vi "CU_RatingVoting.vi"(8 "Classification Distribution":i32[][][](array[numeric]), 11 "IndicatorMatrix":dbl[][](array[numeric])) -> (3 "Class Index":i32)   [LabVIEW 2016, in "Classifier.lvlib"]
uses:
  <vilib>/Analysis/baseanly.llb/A x Vector.vi
  Classifier.lvlib
  <vilib>/Analysis/NI_AALBase.lvlib
panel:
  # "This VI is a part of BCI Design library, http://www.ru-bci.org \nCopyright © 2020, Sotnikov Peter, All rights reserved. License: CC BY-NC 4.0"
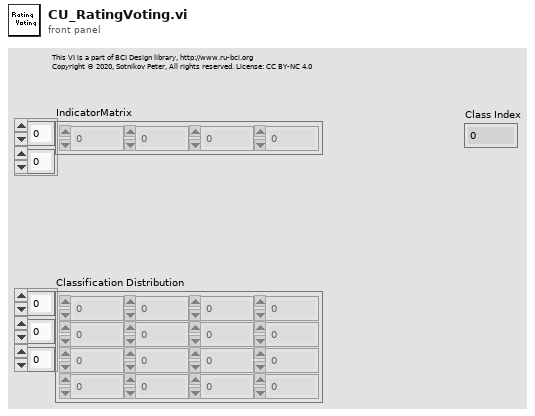
[diagram p1: front panel]
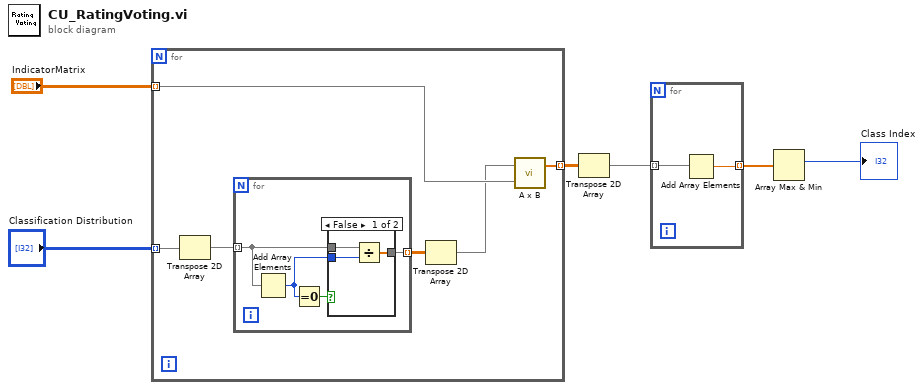
[diagram p0: block diagram]
diagram:
  n1 = for {
    tunnel: "IndicatorMatrix" -> [w12] mode=indexing
    tunnel: [w11] -> w5 mode=indexing
    tunnel: "Classification Distribution" -> [w10] mode=indexing
    n2 = Transpose 2D Array(2D array=w10) -> (transposed array=w9:i32[][])
    n3 = for {
      tunnel: w9 -> [w16] mode=indexing
      tunnel: [w15] -> w8 mode=indexing
      n4 = Add Array Elements(numeric array=w16) -> (sum=w13:i32)
      n5 = Equal To 0?(x=w13) -> (x = 0?=w14:bool)
      n6 = case shown="False" w14 {
        tunnel: w16 -> [w19 w20]
        tunnel: w13 -> [w18 _]
        tunnel: [w17 w20] -> w15
        frame False {
          n7 = Divide(x=w19, y=w18) -> (x/y=w17:dbl[])
        }
        frame True {
        }
      }
    }
    n8 = Transpose 2D Array(2D array=w8) -> (transposed array=w7:dbl[][])
    n9 = call-poly <vilib>:"A x B.vi"("Vector"=w12, "A"=w7) -> ("A x Vector"=w11:dbl[])  [unwired: 1 out]
  }
  n10 = Transpose 2D Array(2D array=w5) -> (transposed array=w4:dbl[][])
  n11 = for {
    tunnel: w4 -> [w22] mode=indexing
    tunnel: [w21] -> w3 mode=indexing
    n12 = Add Array Elements(numeric array=w22) -> (sum=w21:dbl)
  }
  n13 = Array Max & Min(array=w3) -> (max index (indices)=→"Class Index":i32)  [unwired: 3 out]
